vi "get_usernames.vi"(2 "error in (no error)":errorcluster) -> (0 "error out":errorcluster, 1 "UserID output":string[](array[string]))   [LabVIEW 2009]
uses:
  <vilib>/addons/database/Connection.llb/DB Tools Open Connec (String).vi
  DB_Info.vi
  <vilib>/addons/database/_DB Variant To Data/Database Variant To Data.xnode
  <vilib>/addons/database/NI_Database_API.lvlib
panel:
  out "UserID Drop-down":string(combo)
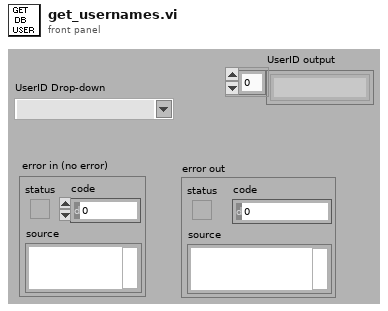
[diagram p1: front panel]
types:
  T1 = typedef "NI_Database_API.lvlib/Conn ObjectReference.ctl" = refnum<k1>
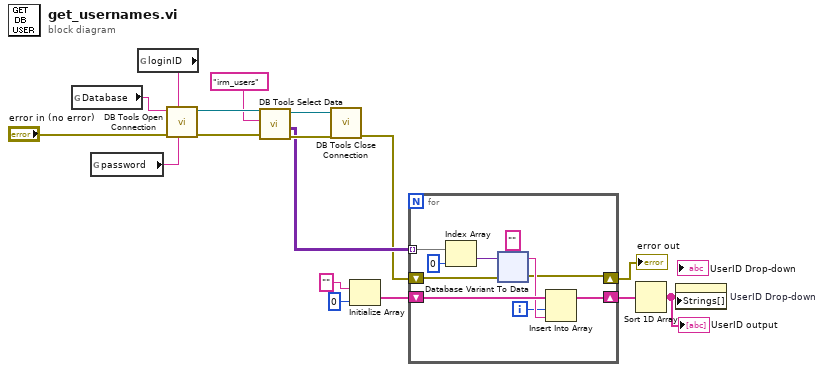
[diagram p0: block diagram]
diagram:
  n1 = global read "DB_Info.vi" "Database"() -> (w2:string)
  n2 = global read "DB_Info.vi" "password"() -> (w1:string)
  n3 = global read "DB_Info.vi" "loginID"() -> (w17:string)
  n4 = call-poly <vilib>:"DB Tools Open Connection.vi"("password"=w1, "userID"=w17, "error in (no error)"="error in (no error)", "connection information"=w2) -> ("error out"=w15:errorcluster, "connection reference"=w14:T1)  [unwired: 1 in, 3 out]
  n5 = call <vilib>:"DB Tools Select Data.vi"("error in (no error)"=w15, "table"="irm_users", "connection reference"=w14) -> ("error out"=w11:errorcluster, "data"=w7:variant[][], "connection reference out"=w12:T1)  [unwired: 1 in, 2 out]
  n6 = call <vilib>:"DB Tools Close Connection.vi"("error in (no error)"=w11, "connection reference"=w12) -> ("error out"=w6:errorcluster)  [unwired: 5 out]
  n7 = Initialize Array("" ("userID"), 0 ("dimension size")) -> (w8:string[])
  n8 = for {
    shift-right: [w22] -> w4
    shift-left: w8 -> [w24]
    tunnel: w7 -> [w26] mode=indexing
    shift-right: [w20] -> w5
    shift-left: w6 -> [w21]
    i -> [w18]
    n9 = Index Array(array=w26, index=0 ("disabled index (col)")) -> (element=w25:variant)
    n10 = xnode "Database Variant To Data"("database variant"=w25, "error in"=w21, "type"="" ("userID")) -> ("data"=w23:string, "error out"=w20:errorcluster)
    n11 = Insert Into Array(array=w24, index=w18, new element=w23) -> (w22:string[])
  }
  "error out" <- w5
  n12 = Sort 1D Array(array=w4) -> (sorted array=w3:string[])
  "UserID output" <- w3
  n13 = property on="UserID Drop-down" class="CmbBox"("Strings[]"=w3) -> ()  [unwired: 2 in, 2 out]
